vi "sub_zoom-synch.vi"(10 "gmap info out":T1) -> ()   [LabVIEW 2019]
uses:
  gmap_info.ctl
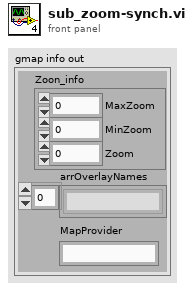
[diagram p1: front panel]
types:
  T1 = typedef "gmap_info.ctl" = cluster{"Zoon_info":cluster{"MaxZoom":dbl, "MinZoom":dbl, "Zoom":dbl}, "arrOverlayNames":string[], "MapProvider":string}
  T2 = cluster{"VLP16 cfg":refnum<vi>, "TIM571 cfg":refnum<vi>, "PID cfg":refnum<vi>, "AGV cfg":refnum<vi>, "GPS cfg":refnum<vi>, "camera cfg":refnum<vi>, "ybbaek copyright":refnum<vi>, "Obstacle limit cfg":refnum<vi>, "State machine cfg":refnum<vi>, "Lookahead cfg":refnum<vi>, "waypoint files cfg":refnum<vi>, "Vison cfg":refnum<vi>, "RPLidar cfg":refnum<vi>, "point all":refnum<vi>, "HW info":refnum<vi>}
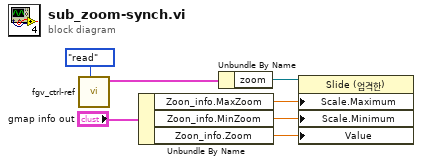
[diagram p0: block diagram]
diagram:
  n1 = call "fgv_ctrl-ref.vi"("cmd"=enum16{"read", "write"}."read") -> ("ref out"=w6:T2)  [unwired: 9 in, 1 out]
  n2 = Unbundle By Name("gmap info out") -> ("Zoon_info.MaxZoom"=w1:dbl, "Zoon_info.MinZoom"=w2:dbl, "Zoon_info.Zoom"=w3:dbl)
  n3 = Unbundle By Name(w6) -> ("zoom"=w7:refnum<vi>)
  n4 = property on="프로퍼티 노드" class="Slide (엄격한)"(reference=w7, "Scale.Maximum"=w1, "Scale.Minimum"=w2, "Value"=w3) -> ()  [unwired: 1 in, 2 out]
